vi "Init.vi"(8 "error in (no error)":errorcluster, 11 "Ni-Scope Digitizer in":refnum<class "Ni-Scope Digitizer.lvclass">) -> (0 "error out":errorcluster, 3 "Ni-Scope Digitizer out":refnum<class "Ni-Scope Digitizer.lvclass">)   [LabVIEW 2015, in "Ni-Scope Digitizer.lvclass"]
uses:
  Ni-Scope Digitizer.lvclass
  <instrlib>/niScope/Configure/Trigger/niScope Configure Trigger Digital.vi
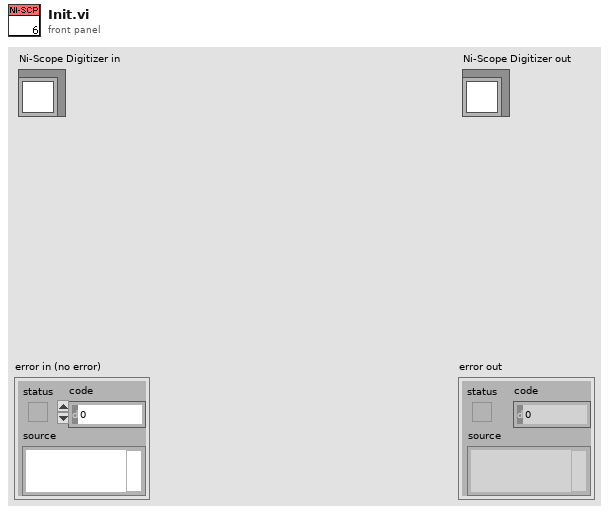
[diagram p1: front panel]
types:
  T1 = typedef "niScope trigger source digital.ctl" = string
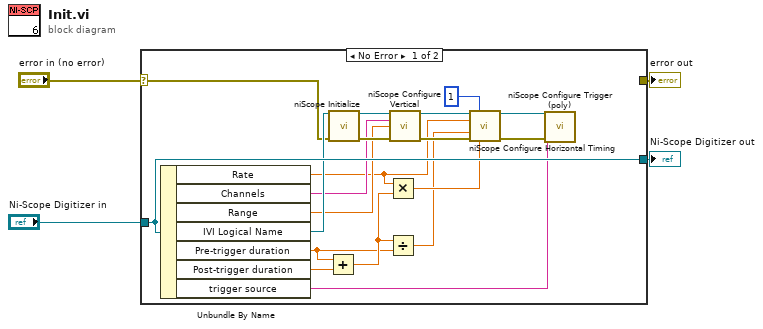
[diagram p0: block diagram]
diagram:
  n1 = case shown="No Error" "error in (no error)" {
    selector: "error in (no error)" -> [w21 w25]
    tunnel: [_ w25] -> w3
    tunnel: [w23 w24] -> w1
    tunnel: "Ni-Scope Digitizer in" -> [w23 w24]
    frame No Error {
      n2 = Unbundle By Name(w23) -> ("Rate"=w12:dbl, "Channels"=w17:string, "Range"=w18:dbl, "IVI Logical Name"=w22:refnum<k15>, "Pre-trigger duration"=w9:dbl, "Post-trigger duration"=w13:dbl, "trigger source"=w5:T1)
      n3 = Add(x=w9, y=w13) -> (x+y=w10:dbl)
      n4 = call <instrlib>:"niScope Initialize.vi"("resource name"=w22, "error in"=w21) -> ("instrument handle"=w19:refnum<k15>, "error out"=w20:errorcluster)  [unwired: 2 in, 10 out]
      n5 = Multiply(x=w12, y=w10) -> (x*y=w11:dbl)
      n6 = Divide(x=w10, y=w9) -> (x/y=w8:dbl)
      n7 = call <instrlib>:"niScope Configure Vertical.vi"("instrument handle"=w19, "channels"=w17, "vertical range"=w18, "error in"=w20) -> ("instrument handle out"=w15:refnum<k15>, "error out"=w16:errorcluster)  [unwired: 10 in]
      n8 = call <instrlib>:"niScope Configure Horizontal Timing.vi"("instrument handle"=w15, "number of records"=1, "min sample rate"=w12, "reference position"=w8, "error in"=w16, "min record length"=w11) -> ("instrument handle out"=w7:refnum<k15>, "error out"=w6:errorcluster)  [unwired: 1 in, 7 out]
      n9 = call-poly <instrlib>:"niScope Configure Trigger (poly).vi"("instrument handle"=w7, "trigger source"=w5, "error in"=w6) -> ()  [unwired: 4 in, 9 out]
    }
    frame Error {
    }
  }
  "error out" <- w3
  "Ni-Scope Digitizer out" <- w1
